vi "DiscoverTypeDefs.vi"(8 "Error In":errorcluster, 11 "Application Reference":refnum<vi>) -> (0 "Error Out":errorcluster, 2 "CtrlType Counts":T1, 3 "All Controls":T2(array[cluster]))   [LabVIEW 2013]
doc: "Looks at all VIs in memory, belonging to the specified Application Instance, and lists all VIs of type \"Control\" (i.e. having a .ctl extension). Each is tagged as being either a normal control, a normal Type Def control, or a Strict Type Def control. Counts for each of these three types are also provided, as well as how many total items (VIs + Controls) from the specifed Application Instance were processed."
uses:
  CtrlVITypeCounts.ctl
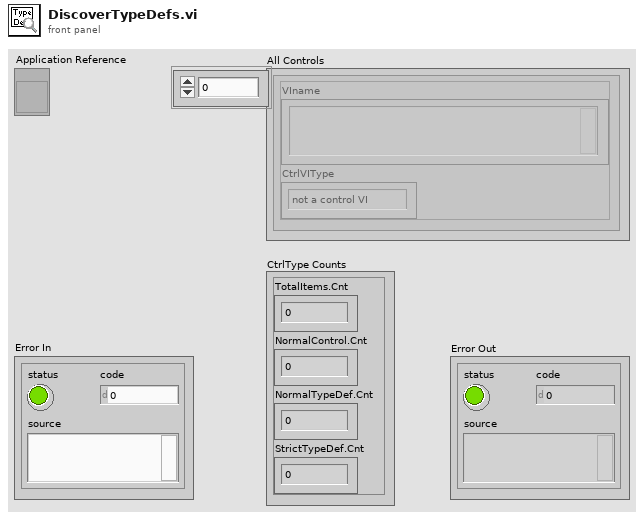
[diagram p1: front panel]
types:
  T1 = typedef "CtrlVITypeCounts.ctl" = cluster{"TotalVIs.Cnt":u32, "NormalControl.Cnt":u32, "NormalTypeDef.Cnt":u32, "StrictTypeDef.Cnt":u32}
  T2 = cluster{"VIname":string, "CtrlVIType":enum32{"not a control VI", "control", "typedef", "strict typedef"}}[]
  T3 = cluster{"VIname":string, "CtrlVIType":enum32{"not a control VI", "control", "typedef", "strict typedef"}}
  T4 = enum32{"not a control VI", "control", "typedef", "strict typedef"}
  T5 = enum32{"invalid VI type", "Standard VI", "Control VI", "Global VI", "Polymorphic VI", "Configuration VI", "SubSystem", "Facade VI", "Method VI", "Statechart Diagram VI"}
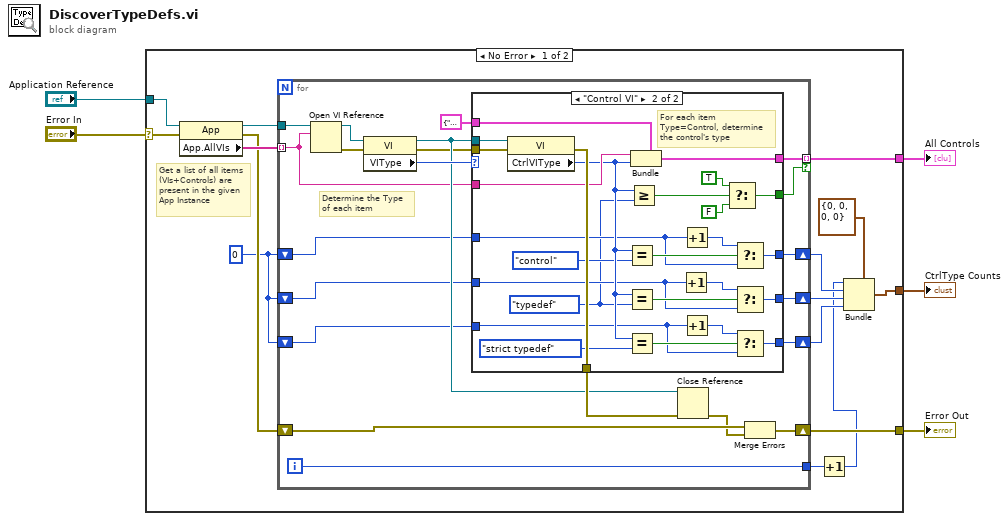
[diagram p0: block diagram]
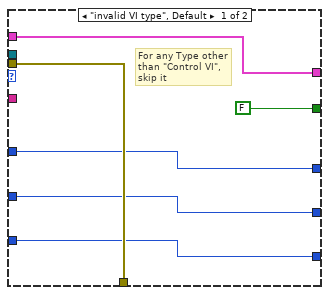
[diagram p2: hidden frame]
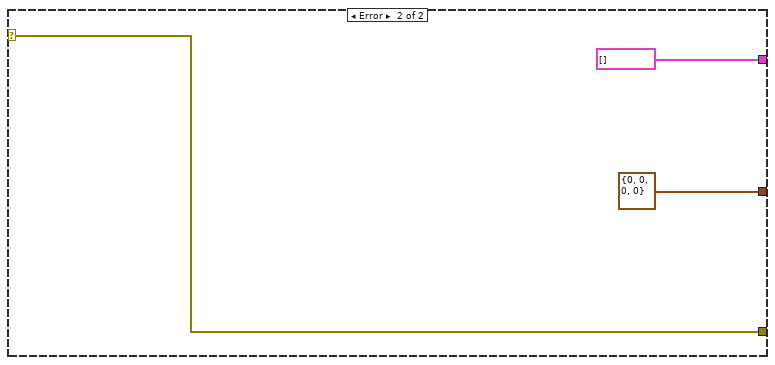
[diagram p3: hidden frame]
diagram:
  n1 = case shown="No Error" "Error In" {
    selector: "Error In" -> [w19 w76]
    tunnel: [w20 w76] -> w5
    tunnel: "Application Reference" -> [w16 _]
    tunnel: [w15 T2 []] -> w2
    tunnel: [w12 T1 {"TotalVIs.Cnt"=0, "NormalControl.Cnt"=0, "NormalTypeDef.Cnt"=0, "StrictTypeDef.Cnt"=0} ("CtrlVIType Counts")] -> w1
    frame No Error {
      w13 = u32 0
      # "Get a list of all items \n(VIs+Controls) are present in the given App Instance"
      n2 = property class="App"(reference=w16, error in=w19) -> (reference out=w18:refnum<vi>, error out=w14:errorcluster, "App.AllVIs"=w17:string[])
      n3 = for {
        tunnel: w17 -> [w29] mode=indexing
        shift-right: [w37] -> w20
        shift-left: w14 -> [w39]
        tunnel: w18 -> [w36]
        tunnel: [w33] -> w15 mode=indexing if=w30
        shift-right: [w25] -> w9
        shift-left: w13 -> [w22]
        shift-right: [w26] -> w7
        shift-left: w13 -> [w23]
        shift-right: [w27] -> w8
        shift-left: w13 -> [w24]
        tunnel: [w21] -> w10
        i -> [w21]
        # "Determine the Type \nof each item"
        n4 = Open VI Reference(application reference (local)=w36, vi path=w29) -> (vi reference=w41:refnum<vi>, error out=w40:errorcluster)  [unwired: 4 in]
        n5 = property class="VI"(reference=w41, error in=w40) -> (reference out=w32:refnum<vi>, error out=w31:errorcluster, "VIType"=w35:T5)
        n6 = case shown="\"Control VI\"" w35 {
          tunnel: [w47 w73] -> w34
          tunnel: w32 -> [_ w72]
          tunnel: [w45 w70] -> w33
          tunnel: w31 -> [w47 w71]
          tunnel: [FALSE w65] -> w30
          tunnel: w29 -> [_ w69]
          tunnel: T3 {"VIname"="", "CtrlVIType"=enum."not a control VI"} ("Cluster") -> [w45 w68]
          tunnel: [w42 w56] -> w27
          tunnel: [w43 w55] -> w26
          tunnel: [w44 w54] -> w25
          tunnel: w24 -> [w42 w49]
          tunnel: w23 -> [w43 w50]
          tunnel: w22 -> [w44 w51]
          frame "invalid VI type", Default {
            # "For any Type other \nthan \"Control VI\", \nskip it"
          }
          frame "Control VI" {
            w48 = T4."typedef" ("Control VI Type")
            # "For each item \nType=Control, determine\nthe control's type"
            n7 = property class="VI"(reference=w72, error in=w71) -> (error out=w73:errorcluster, "CtrlVIType"=w63:T4)  [unwired: 1 out]
            n8 = Equal?(x=w63, y=T4."control" ("Control VI Type")) -> (x = y?=w60:bool)
            n9 = Equal?(x=w63, y=w48) -> (x = y?=w59:bool)
            n10 = Equal?(x=w63, y=T4."strict typedef" ("Control VI Type")) -> (x = y?=w58:bool)
            n11 = Greater Or Equal?(x=w63, y=w48) -> (x >= y?=w64:bool)
            n12 = Bundle(cluster=w68, "VIname"=w69, "CtrlVIType"=w63) -> (w70:T3)
            n13 = Increment(x=w50) -> (x+1=w53:u32)
            n14 = Increment(x=w51) -> (x+1=w52:u32)
            n15 = Increment(x=w49) -> (x+1=w57:u32)
            n16 = Select(t=TRUE, s=w64, f=FALSE) -> (s? t:f=w65:bool)
            n17 = Select(t=w52, s=w60, f=w51) -> (s? t:f=w54:u32)
            n18 = Select(t=w53, s=w59, f=w50) -> (s? t:f=w55:u32)
            n19 = Select(t=w57, s=w58, f=w49) -> (s? t:f=w56:u32)
          }
        }
        n20 = Close Reference(reference=w32, error in (no error)=w34) -> (error out=w38:errorcluster)
        n21 = Merge Errors(w39, w38) -> (w37:errorcluster)
      }
      n22 = Increment(x=w10) -> (x+1=w6:i32)
      n23 = Bundle(cluster=T1 {"TotalVIs.Cnt"=0, "NormalControl.Cnt"=0, "NormalTypeDef.Cnt"=0, "StrictTypeDef.Cnt"=0} ("CtrlVIType Counts"), "TotalVIs.Cnt"=w6, "NormalControl.Cnt"=w9, "NormalTypeDef.Cnt"=w7, "StrictTypeDef.Cnt"=w8) -> (w12:T1)
    }
    frame Error {
    }
  }
  "Error Out" <- w5
  "All Controls" <- w2
  "CtrlType Counts" <- w1
